vi "Inject Attribute List.vi"(6 "Attributes Ref":refnum<data-value>, 8 "error in (no error)":errorcluster, 11 "Stop High Pressure Wash in":refnum<class "Stop High Pressure Wash.lvclass">) -> (0 "error out":errorcluster, 3 "Stop High Pressure Wash out":refnum<class "Stop High Pressure Wash.lvclass">)   [LabVIEW 2019, in "Stop High Pressure Wash.lvclass"]
uses:
  <vilib>/gpm_packages/@cs/Car-wash/Source/Process Steps/Stop High Pressure Wash/Stop High Pressure Wash.lvclass
  <vilib>/gpm_packages/@cs/lookup-table/Source/LookupTable/LookupTable.lvclass
  <vilib>/gpm_packages/@cs/lookup-table/Source/LookupTable/LookupTable.lvclass/LookupTable.ctl
  <vilib>/gpm_packages/@cs/Car-wash/Source/Process Steps/Stop High Pressure Wash/Stop High Pressure Wash.lvclass/Stop High Pressure Wash.ctl
  c4f79ea2-7aa7-41a7-87af-50bb2e8807d3.vi
  <vilib>/gpm_packages/@cs/lookup-table/Source/LookupTable/Read Table Reference.vi
  c4f79ea2-7aa7-41a7-87af-50bb2e8807d3.vi/072e2c9f-2285-40ae-ba24-b92b504194f8.vi
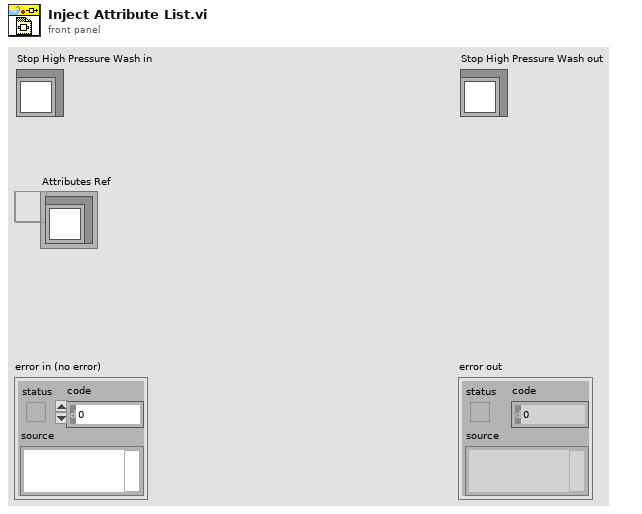
[diagram p1: front panel]
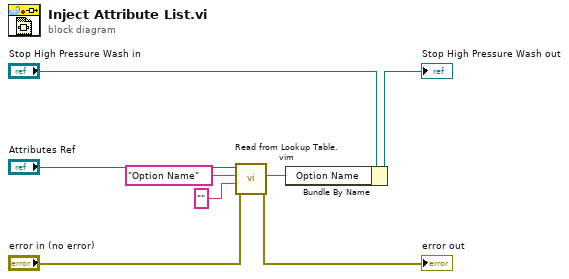
[diagram p0: block diagram]
diagram:
  n1 = call "Read from Lookup Table.vim"("error in (no error)"="error in (no error)", "Type"="", "Item Name"="Option Name", "LookupTable Reference"="Attributes Ref") -> ("error out"=→"error out":errorcluster, "Value"=w6:string)  [unwired: 4 in, 2 out]
  n2 = Bundle By Name(cluster="Stop High Pressure Wash in", "Option Name"=w6) -> (→"Stop High Pressure Wash out":refnum<class "Stop High Pressure Wash.lvclass">)
